vi "speed.vi"(10 "motor in":dbl, 11 "motor 1":dbl) -> (3 "Numeric":dbl)   [LabVIEW 2017]
uses:
  Global pulses.vi
panel:
  out "Enum":T1(ring)
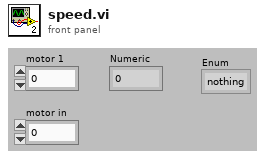
[diagram p1: front panel]
types:
  T1 = enum16{"nothing", "high speed", "medium speed", "low speed"}
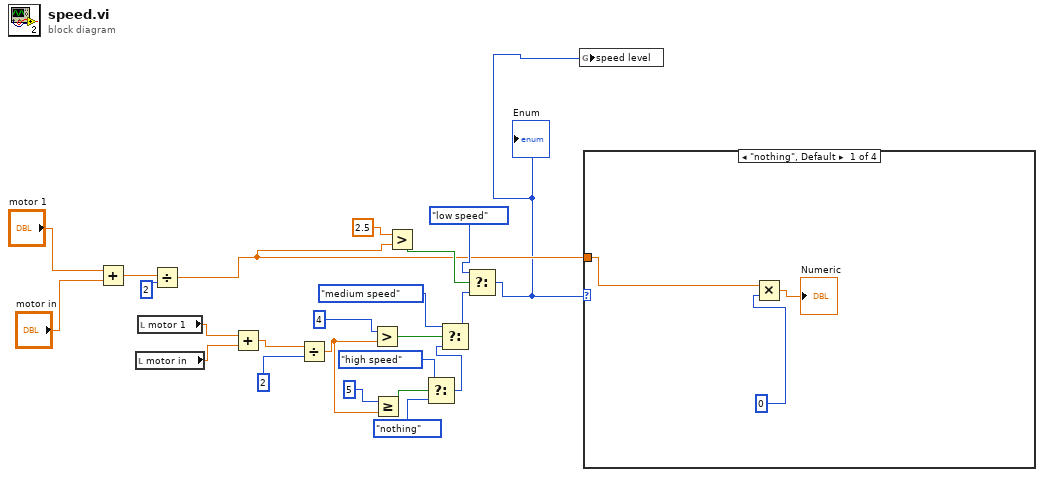
[diagram p0: block diagram]
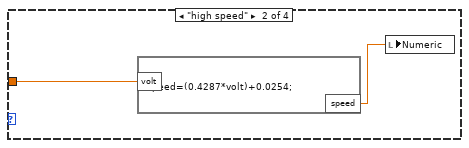
[diagram p2: hidden frame]
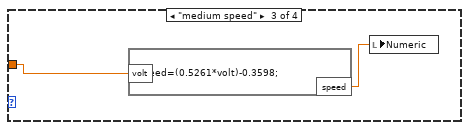
[diagram p3: hidden frame]
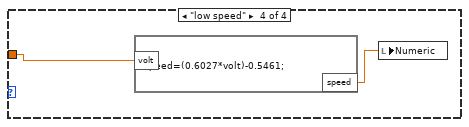
[diagram p4: hidden frame]
diagram:
  n1 = Add(x="motor 1", y="motor in") -> (x+y=w20:dbl)
  n2 = local read "motor in"() -> (w14:dbl)
  n3 = local read "motor 1"() -> (w15:dbl)
  n4 = Divide(x=w20, y=2) -> (x/y=w5:dbl)
  n5 = Add(x=w15, y=w14) -> (x+y=w13:dbl)
  n6 = Divide(x=w13, y=2) -> (x/y=w3:dbl)
  n7 = Greater?(x=4, y=w3) -> (0:w6:bool)
  n8 = Greater Or Equal?(x=5, y=w3) -> (x >= y?=w2:bool)
  n9 = Greater?(x=2.5, y=w5) -> (0:w18:bool)
  n10 = Select(t=T1."high speed", s=w2, f=T1."nothing") -> (s? t:f=w10:T1)
  n11 = Select(t=T1."medium speed", s=w6, f=w10) -> (s? t:f=w16:T1)
  n12 = Select(t=T1."low speed", s=w18, f=w16) -> (s? t:f=w1:T1)
  "Enum" <- w1
  n13 = global write "Global pulses.vi" "speed level"(w1) -> ()
  n14 = case shown="\"nothing\", Default" w1 {
    tunnel: w5 -> [w25 w28 w30 w32]
    frame "nothing", Default {
      n15 = Multiply(x=w25, y=0) -> (x*y=→"Numeric":dbl)
    }
    frame "high speed" {
      n16 = formula code="speed=(0.4287*volt)+0.0254;"("volt"=w28) -> ("speed"=w27:dbl)
      n17 = local write "Numeric"(w27) -> ()
    }
    frame "medium speed" {
      n18 = formula code="speed=(0.5261*volt)-0.3598;"("volt"=w30) -> ("speed"=w29:dbl)
      n19 = local write "Numeric"(w29) -> ()
    }
    frame "low speed" {
      n20 = formula code="speed=(0.6027*volt)-0.5461;"("volt"=w32) -> ("speed"=w31:dbl)
      n21 = local write "Numeric"(w31) -> ()
    }
  }
